vi "Seq Set Process Print LabCode.vi"(8 "Segment Data":T1) -> (0 "Step Hisitory":string[](array[string]), 2 "Segment Data 2":T1)   [LabVIEW 2015]
uses:
  Sequence/type defs/Sequence Info.ctl
  type defs/Process Print LabCode.ctl
panel:
  in  "Fixed code":string
  in  "Label file path":path
  out "String 2":string="Pre Run Station - Glass - Vent Open"
  out "error out":errorcluster
  in  "Description":string
  in  "Save":bool
  in  "Cancel":bool
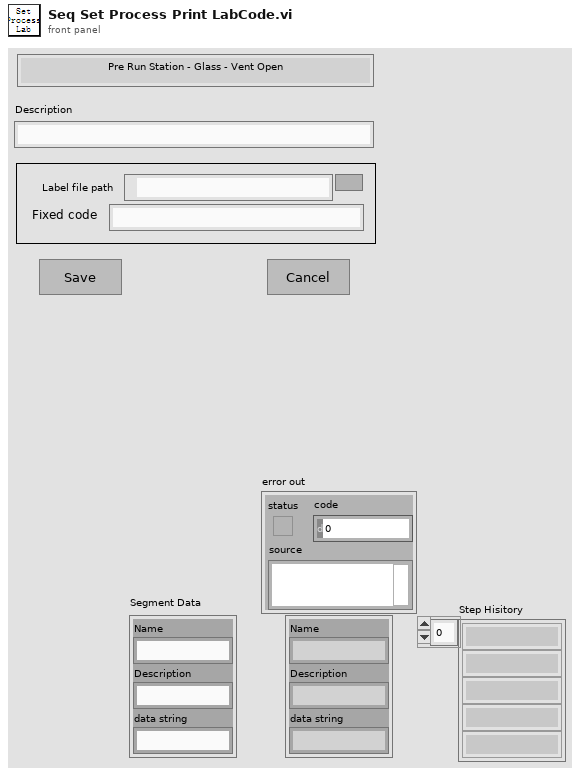
[diagram p1: front panel]
types:
  T1 = typedef "Sequence Info.ctl" = cluster{"Name":string, "Description":string, "data string":string}
  T2 = typedef "Process Print LabCode.ctl" = cluster{"Label file path":path, "Fixed code":string}
  T3 = cluster{"Segment Data":T1, "Process Print LabCode":T2, "Old Data":string, "New Data":string}
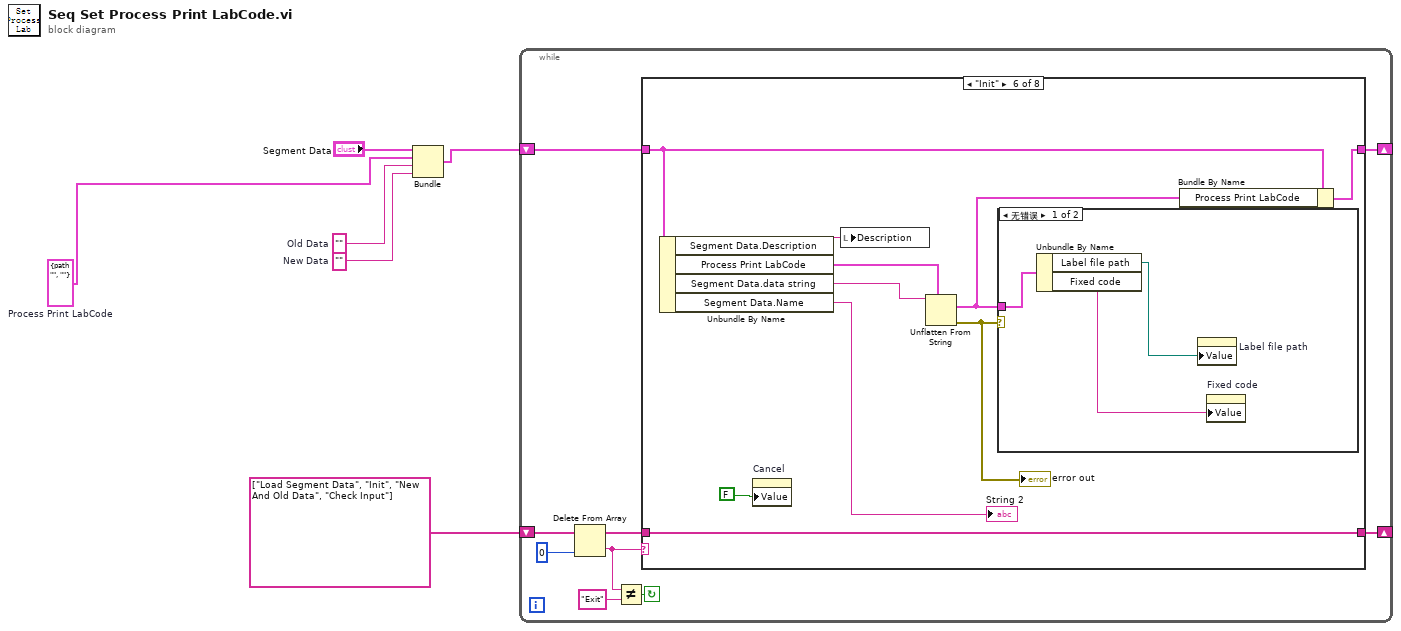
[diagram p0: block diagram]
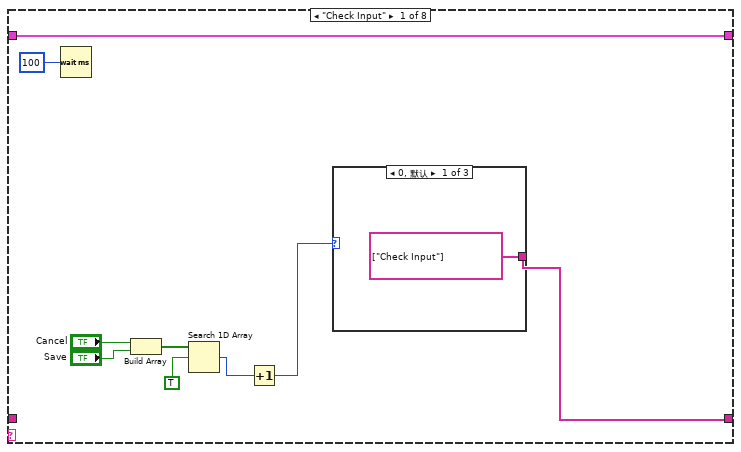
[diagram p2: hidden frame]
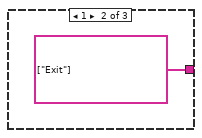
[diagram p3: hidden frame]
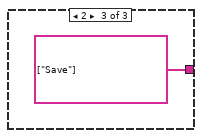
[diagram p4: hidden frame]
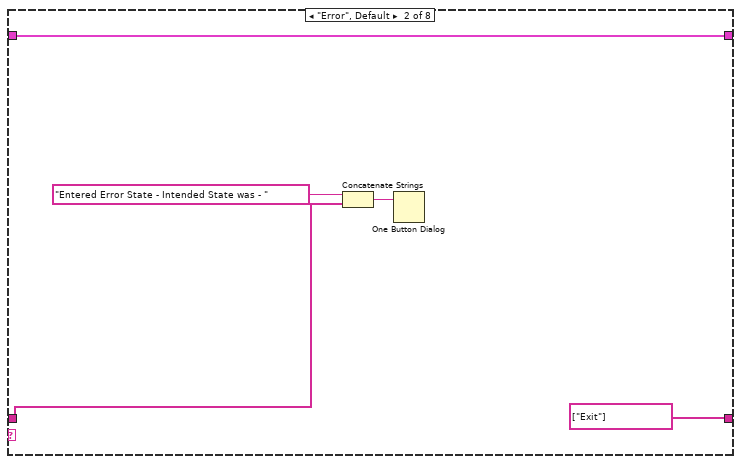
[diagram p5: hidden frame]
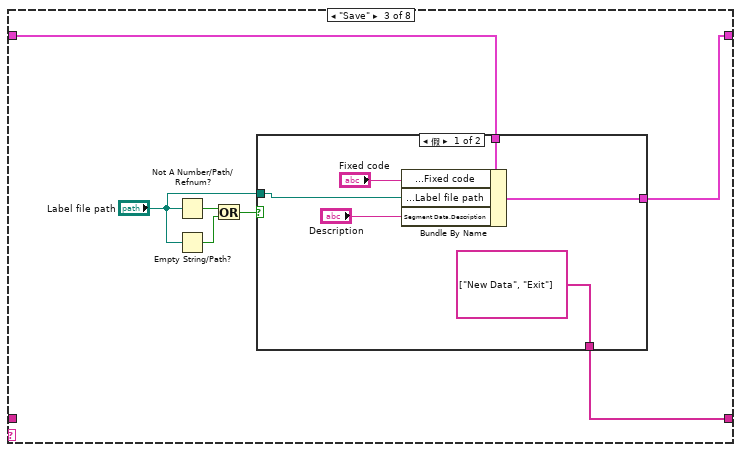
[diagram p6: hidden frame]
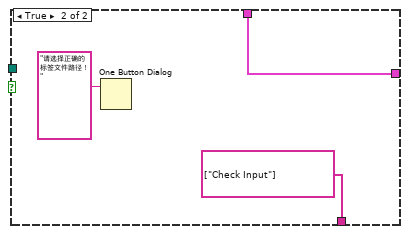
[diagram p7: hidden frame]
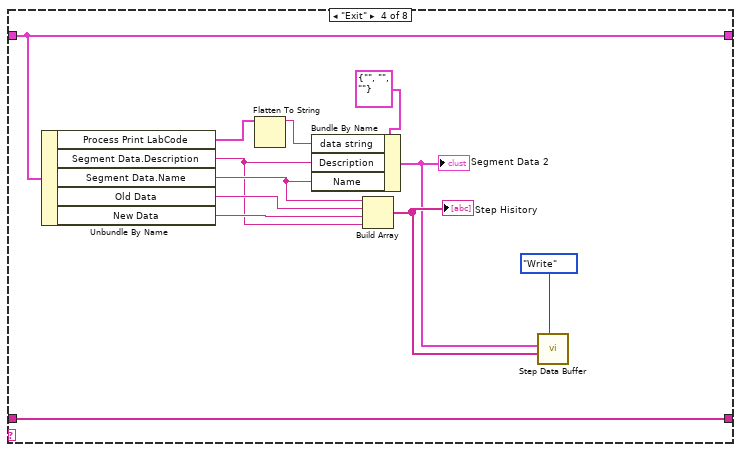
[diagram p8: hidden frame]
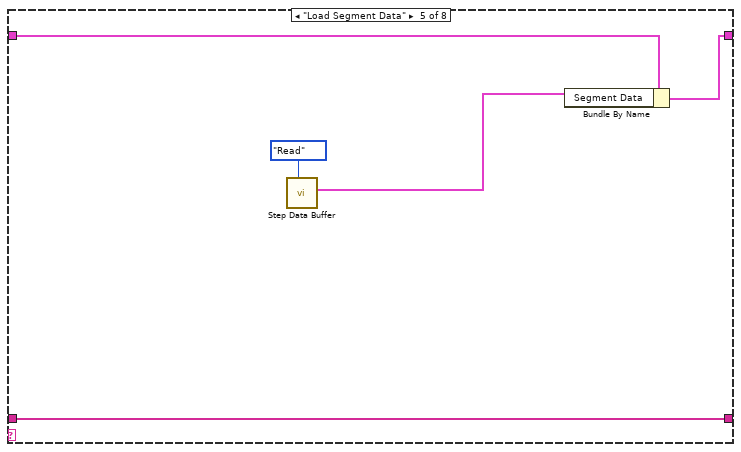
[diagram p9: hidden frame]
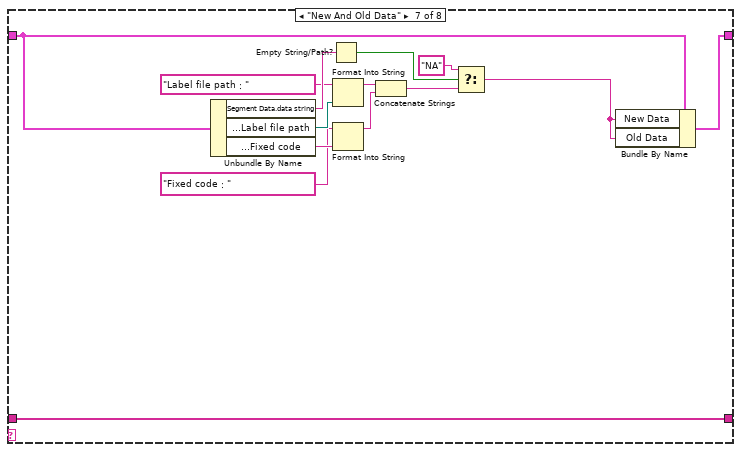
[diagram p11: hidden frame]
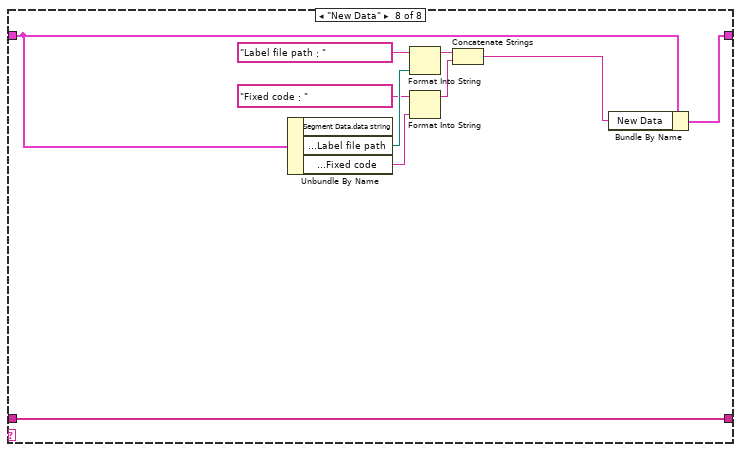
[diagram p12: hidden frame]
diagram:
  w1 = T2 {"Label file path"=path "", "Fixed code"=""}  # Process Print LabCode
  w3 = ""  # New Data
  w4 = ""  # Old Data
  n1 = Bundle("Segment Data"="Segment Data", "Process Print LabCode"=w1, "Old Data"=w4, "New Data"=w3) -> (w5:T3)  [unwired: 1 in]
  n2 = while {
    shift-right: [w15] -> _
    shift-left: string[] ["Load Segment Data", "Init", "New And Old Data", "Check Input"] ("Event queue out") -> [w11]
    shift-right: [w13] -> _
    shift-left: w5 -> [w14]
    stop <- w7 continue-if-true
    n3 = Delete From Array(array=w11, index=0 ("Index")) -> (deleted portion=w9:string, array with subset deleted=w10:string[])  [unwired: 1 in]
    n4 = Not Equal?(x=w9, y="Exit" ("Exit Event")) -> (x != y?=w7:bool)
    n5 = case shown="\"Init\"" w9 {
      tunnel: w10 -> [_ w29 _ w60 w65 w75 w92 w101]
      tunnel: [w16 string[] ["Exit"] ("event queue out") w39 w60 w65 w75 w92 w101] -> w15
      tunnel: w14 -> [w19 w32 w38 w53 w62 w68 w85 w100]
      tunnel: [w19 w32 w37 w53 w61 w67 w84 w99] -> w13
      frame "Check Input" {
        n6 = Wait (ms)(milliseconds to wait=u32 100) -> ()  [unwired: 1 out]
        n7 = Build Array("Cancel", "Save") -> (w21:bool[])
        n8 = Search 1D Array(1D array=w21, element=TRUE) -> (index of element=w17:i32)  [unwired: 1 in]
        n9 = Increment(x=w17) -> (x+1=w18:i32)
        n10 = case shown="0, 默认" w18 {
          tunnel: [string[] ["Check Input"] ("Events to Insert") string[] ["Exit"] ("Events to Insert") string[] ["Save"] ("Events to Insert")] -> w16
          frame 0, Default {
          }
          frame 1 {
          }
          frame 2 {
          }
        }
      }
      frame "Error", Default {
        n11 = Concatenate Strings("Entered Error State - Intended State was - " ("string"), w29) -> (w30:string)
        n12 = One Button Dialog(message=w30) -> ()  [unwired: 1 in, 1 out]
      }
      frame "Save" {
        n13 = Not A Number/Path/Refnum?(number/path/refnum="Label file path") -> (NaN/Path/Refnum?=w35:bool)
        n14 = Empty String/Path?(string/path="Label file path") -> (empty?=w33:bool)
        n15 = Or(x=w35, y=w33) -> (x .or. y?=w34:bool)
        n16 = case shown="假" w34 {
          tunnel: [string[] ["New Data", "Exit"] ("Event queue out") string[] ["Check Input"] ("Events to Insert")] -> w39
          tunnel: w38 -> [w44 w46]
          tunnel: "Label file path" -> [w42 _]
          tunnel: [w41 w46] -> w37
          frame False {
            n17 = Bundle By Name(cluster=w44, "Process Print LabCode.Fixed code"="Fixed code", "Process Print LabCode.Label file path"=w42, "Segment Data.Description"="Description") -> (w41:T3)
          }
          frame True {
            n18 = One Button Dialog(message="请选择正确的标签文件路径！" ("消息")) -> ()  [unwired: 1 in, 1 out]
          }
        }
      }
      frame "Exit" {
        n19 = Unbundle By Name(w53) -> ("Process Print LabCode"=w59:T2, "Segment Data.Description"=w49:string, "Segment Data.Name"=w54:string, "Old Data"=w56:string, "New Data"=w55:string)
        n20 = Flatten To String(anything=w59) -> (data string=w57:string)  [unwired: 3 in, 2 out]
        n21 = Bundle By Name(cluster=T1 {"Name"="", "Description"="", "data string"=""} ("Segment Data"), "data string"=w57, "Description"=w49, "Name"=w54) -> (w50:T1)
        "Segment Data 2" <- w50
        n22 = Build Array(w54, w56, w55, w49) -> (w51:string[])
        "Step Hisitory" <- w51
        n23 = call "Step Data Buffer.vi"("Mode"=enum16{"Init", "Read", "Write"}."Write", "Step Hisitory In"=w51, "Segment Data"=w50) -> ()  [unwired: 4 in, 5 out]
      }
      frame "Load Segment Data" {
        n24 = call "Step Data Buffer.vi"("Mode"=enum16{"Init", "Read", "Write"}."Read") -> ("Segment Data"=w63:T1)  [unwired: 6 in, 4 out]
        n25 = Bundle By Name(cluster=w62, "Segment Data"=w63) -> (w61:T3)
      }
      frame "Init" {
        n26 = Unbundle By Name(w68) -> ("Segment Data.Description"=w70:string, "Process Print LabCode"=w73:T2, "Segment Data.data string"=w74:string, "Segment Data.Name"=→"String 2":string)
        n27 = property on="Cancel" class="Bool (严格)"("Value"=FALSE ("Cancel")) -> ()  [unwired: 2 in, 2 out]
        n28 = local write "Description"(w70) -> ()
        n29 = Unflatten From String(type=w73, binary string=w74) -> (value=w69:T2, error out=w72:errorcluster)  [unwired: 3 in, 1 out]
        "error out" <- w72
        n30 = case shown="无错误" w72 {
          tunnel: w69 -> [w78 _]
          frame No Error {
            n31 = Unbundle By Name(w78) -> ("Label file path"=w77:path, "Fixed code"=w76:string)
            n32 = property on="Label file path" class="Path"("Value"=w77) -> ()  [unwired: 2 in, 2 out]
            n33 = property on="Fixed code" class="Str"("Value"=w76) -> ()  [unwired: 2 in, 2 out]
          }
          frame Error {
          }
        }
        n34 = Bundle By Name(cluster=w68, "Process Print LabCode"=w69) -> (w67:T3)
      }
      frame "New And Old Data" {
        n35 = Unbundle By Name(w85) -> ("Segment Data.data string"=w91:string, "Process Print LabCode.Label file path"=w87:path, "Process Print LabCode.Fixed code"=w80:string)
        n36 = Empty String/Path?(string/path=w91) -> (empty?=w90:bool)
        n37 = Format Into String(initial string="Label file path：" ("string"), w87) -> (resulting string=w83:string)  [unwired: 2 in, 1 out]
        n38 = Format Into String(initial string="Fixed code：" ("string"), w80) -> (resulting string=w82:string)  [unwired: 2 in, 1 out]
        n39 = Concatenate Strings(w83, w82) -> (w81:string)
        n40 = Select(t="NA", s=w90, f=w81) -> (s? t:f=w88:string)
        n41 = Bundle By Name(cluster=w85, "New Data"=w88, "Old Data"=w88) -> (w84:T3)
      }
      frame "New Data" {
        n42 = Unbundle By Name(w100) -> ("Process Print LabCode.Label file path"=w102:path, "Process Print LabCode.Fixed code"=w97:string)  [unwired: 1 out]
        n43 = Format Into String(initial string="Label file path：" ("string"), w102) -> (resulting string=w95:string)  [unwired: 2 in, 1 out]
        n44 = Format Into String(initial string="Fixed code：" ("string"), w97) -> (resulting string=w94:string)  [unwired: 2 in, 1 out]
        n45 = Concatenate Strings(w95, w94) -> (w93:string)
        n46 = Bundle By Name(cluster=w100, "New Data"=w93) -> (w99:T3)
      }
    }
  }
